vi "configure.vi"(8 "error in (no error)":errorcluster, 11 "DL090503StimulatorScaffold in":refnum<class "StimulatorAK101022TCP.lvclass">) -> (0 "error out":errorcluster, 3 "DL090503StimulatorScaffold out":refnum<class "StimulatorAK101022TCP.lvclass">)   [LabVIEW 2010, in "StimulatorAK101022TCP.lvclass"]
doc: "The dynamic dispatch version of this VI loads and displays the configuration file associated with the plug-in object. The user modify and save the configuration data."
uses:
  StimulatorAK101022TCP.lvclass
  common/xcontrols/XComponentSpecification/XComponentSpecification/XComponentSpecification.xctl
  StimulatorAK101022TCP.lvclass/StimulatorAK101022TCP.ctl
  common/classes/GenericComponent/GenericComponent/GenericComponent.lvclass
panel:
  in  "stringGenerator spec":T1(xcontrol)
  in  "Port":u16=5000
  in  "Address":string="130.60.53.37"
  out "Configuration":string
  in  "cancel button":bool
  in  "save button":bool
  # "Configure AK101022StimulatorTCP"
  # "StringGenerator component"
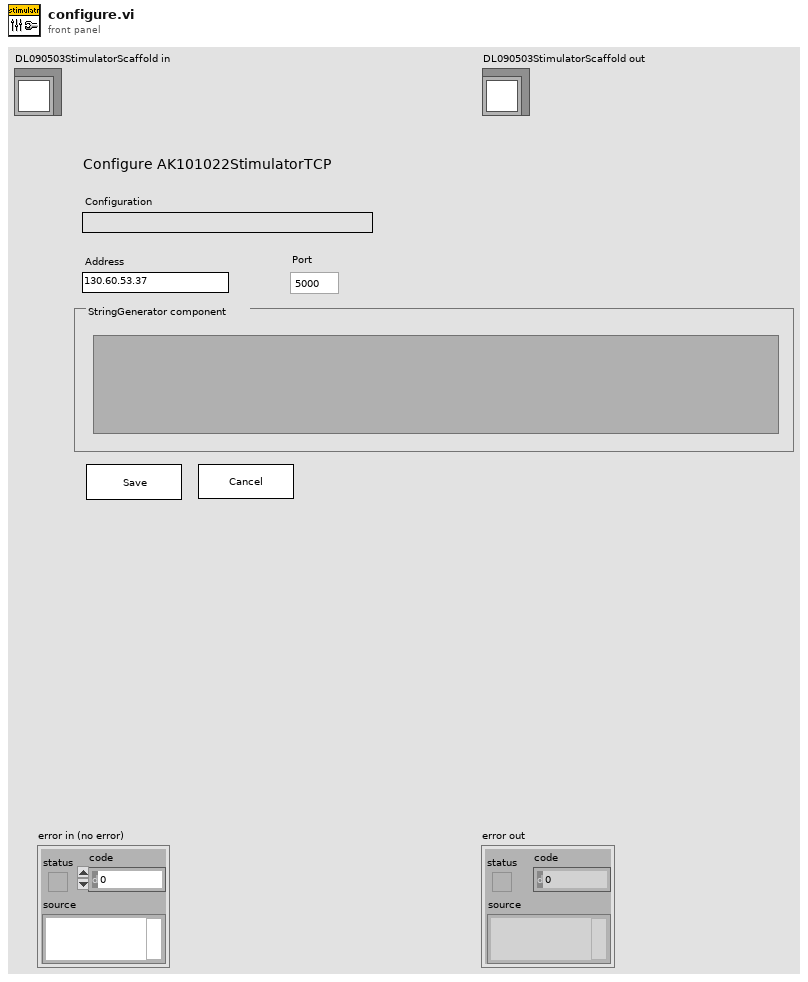
[diagram p1: front panel]
types:
  T1 = cluster{"class path":string, "configuration":string, "label":string, "settings name":string}
  T2 = typedef "plugin_specification.ctl" = cluster{"class path":string, "configuration":string, "label":string, "settings name":string}
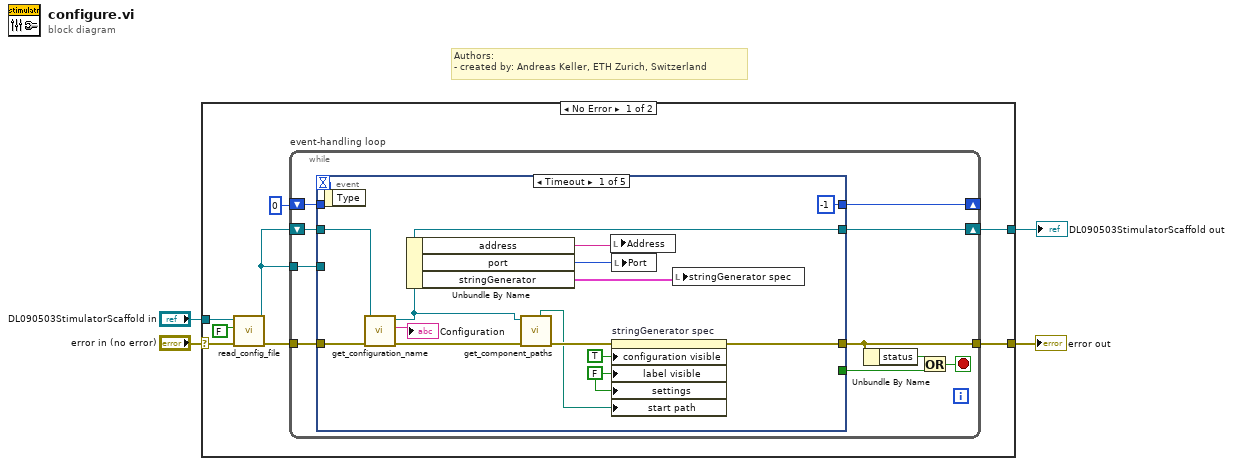
[diagram p0: block diagram]
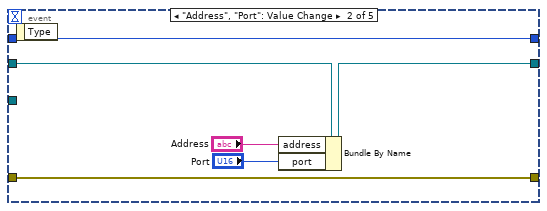
[diagram p2: hidden frame]
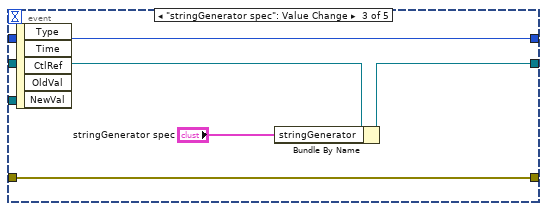
[diagram p3: hidden frame]
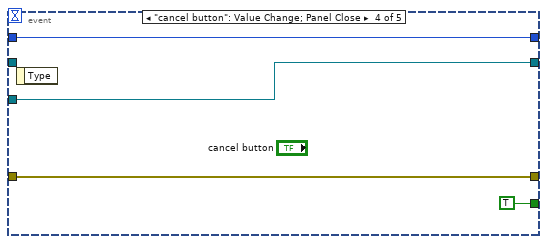
[diagram p4: hidden frame]
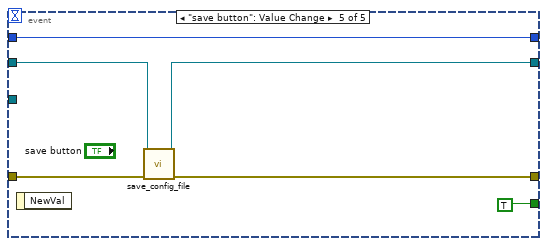
[diagram p5: hidden frame]
diagram:
  # "Authors: \n- created by: Andreas Keller, ETH Zurich, Switzerland"
  n1 = case shown="No Error" "error in (no error)" {
    selector: "error in (no error)" -> [w12 w59]
    tunnel: [w8 w59] -> w4
    tunnel: "DL090503StimulatorScaffold in" -> [w11 w58]
    tunnel: [w7 w58] -> w1
    frame No Error {
      n2 = call-dynamic "read_config_file.vi"("error in (no error)"=w12, "force load?"=FALSE, "GenericPlugin in"=w11) -> ("error out"=w9:errorcluster, "GenericPlugin out"=w5:refnum<class "StimulatorAK101022TCP.lvclass">)  [unwired: 7 in]
      n3 = while "event-handling loop" {
        tunnel: w9 -> [w22]
        tunnel: [w17] -> w8
        shift-right: [w18] -> _
        shift-left: 0 -> [w19]
        shift-right: [w21] -> w7
        shift-left: w5 -> [w20]
        tunnel: w5 -> [w13]
        stop <- w14 stop-if-true
        n4 = event shown="[0] Timeout" {
          selector: _ -> [_ _ _ _ _]
          dyn-events: _ -> [_ _ _ _ _]
          timeout: w19 -> [_ _ _ _ _]
          tunnel: w22 -> [w35 w42 w44 w51 w56]
          tunnel: [w27 w42 w44 w51 w55] -> w17
          tunnel: [w23 w39 w45 w48 w53] -> w21
          tunnel: w20 -> [w36 w40 w46 _ w54]
          tunnel: w19 -> [_ w41 w47 w50 w57]
          tunnel: [-1 w41 w47 w50 w57] -> w18
          tunnel: [_ _ _ TRUE TRUE] -> w16
          tunnel: w13 -> [_ _ _ w48 _]
          event Timeout {
            w24 = FALSE ("label visible")
            n5 = event-data() -> ()  [unwired: 1 in, 1 out]
            n6 = call "get_configuration_name.vi"("error in (no error)"=w35, "GenericPlugin.lvclass in"=w36) -> ("error out"=w30:errorcluster, "configuration name"=→"Configuration":string, "GenericPlugin.lvclass out"=w23:refnum<class "StimulatorAK101022TCP.lvclass">)  [unwired: 7 in]
            n7 = Unbundle By Name(w23) -> ("address"=w32:string, "port"=w31:u16, "stringGenerator"=w29:T2)
            n8 = call-dynamic "get_component_paths.vi"("error in (no error)"=w30, "GenericComponent in"=w23) -> ("error out"=w28:errorcluster, "component type directory"=w26:path)  [unwired: 4 in, 4 out]
            n9 = local write "Address"(w32) -> ()
            n10 = local write "Port"(w31) -> ()
            n11 = property on="stringGenerator spec" class="XComponentSpecification (strict"(error in=w28, "configuration visible"=TRUE, "label visible"=w24, "settings"=w24, "start path"=w26) -> (error out=w27:errorcluster)  [unwired: 1 in, 1 out]
            n12 = local write "stringGenerator spec"(w29) -> ()
          }
          event "Address", "Port": Value Change {
            n13 = event-data() -> ()  [unwired: 1 in, 1 out]
            n14 = Bundle By Name(cluster=w40, "address"="Address", "port"="Port") -> (w39:refnum<class "StimulatorAK101022TCP.lvclass">)
          }
          event "stringGenerator spec": Value Change {
            n15 = event-data() -> ()  [unwired: 1 in, 5 out]
            n16 = Bundle By Name(cluster=w46, "stringGenerator"="stringGenerator spec") -> (w45:refnum<class "StimulatorAK101022TCP.lvclass">)
          }
          event "cancel button": Value Change; Panel Close {
            n17 = event-data() -> ()  [unwired: 1 in, 1 out]
          }
          event "save button": Value Change {
            n18 = event-data() -> ()  [unwired: 1 in, 1 out]
            n19 = call-dynamic "save_config_file.vi"("error in (no error)"=w56, "GenericPlugin in"=w54) -> ("error out"=w55:errorcluster, "GenericPlugin out"=w53:refnum<class "StimulatorAK101022TCP.lvclass">)  [unwired: 8 in]
          }
        }
        n20 = Unbundle By Name(w17) -> ("status"=w15:bool)
        n21 = Or(x=w15, y=w16) -> (x .or. y?=w14:bool)
      }
    }
    frame Error {
    }
  }
  "error out" <- w4
  "DL090503StimulatorScaffold out" <- w1
